vi "Config Sample Clock Rate.vi"(0 "VISA Resource Name":refnum<visa-resource-name>, 5 "Standard (0: IS-95A)":enum16{"IS-95A", "CDMA2000", "WCDMA"}(ring), 7 "Clock Rate (1.0e+8)":dbl=100000000.0 format="%_2e", 11 "error in (no error)":errorcluster {"code" format="%.0x"}) -> (4 "VISA Resource Name Out":refnum<visa-resource-name>, 15 "error out":errorcluster {"code" format="%.0x"})   [LabVIEW 2012, in "Agilent ESG Series.lvlib"]
doc: "This VI sets the sample clock rate for the modulation format.\n\nNotes:\n(1) This VI is valid only on instrument E4438C."
uses:
  <instrlib>/Agilent ESG Series/Agilent ESG Series.lvlib
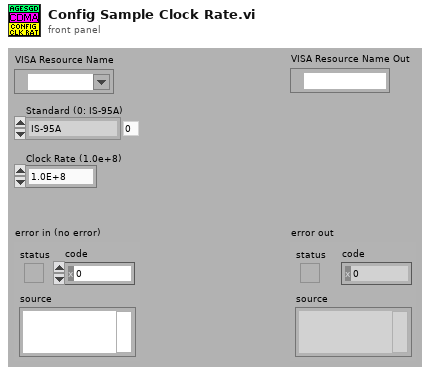
[diagram p1: front panel]
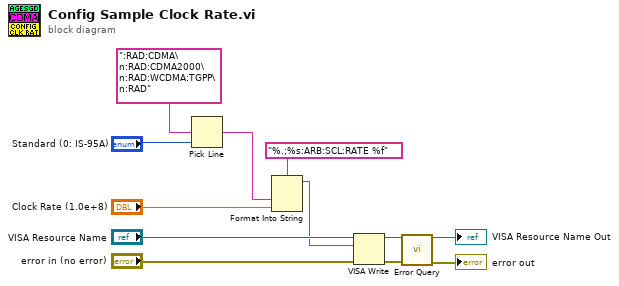
[diagram p0: block diagram]
diagram:
  n1 = Pick Line(multi-line string=":RAD:CDMA\n:RAD:CDMA2000\n:RAD:WCDMA:TGPP\n:RAD", line index="Standard (0: IS-95A)") -> (output string=w5:string)  [unwired: 1 in]
  n2 = Format Into String(format string="%.;%s:ARB:SCL:RATE %f", w5, "Clock Rate (1.0e+8)") -> (resulting string=w1:string)  [unwired: 2 in, 1 out]
  n3 = VISA Write(VISA resource name="VISA Resource Name", write buffer=w1, error in (no error)="error in (no error)") -> (VISA resource name out=w8:refnum<visa-resource-name>, error out=w7:errorcluster)  [unwired: 1 out]
  n4 = call <instrlib>:"Error Query.vi"("VISA Resource Name"=w8, "error in (no error)"=w7) -> ("VISA Resource Name Out"=→"VISA Resource Name Out":refnum<visa-resource-name>, "error out"=→"error out":errorcluster)  [unwired: 10 in, 2 out]
